vi "Save File DOE Reinitialize Drop Downs to Default.vi"(7 "Save Default":enum16{"Standard", "Save To Default"}(ring), 8 "error in (no error)":errorcluster, 11 "Standard Path":path=path "C:/GE/Washer DOE/WasherDOEConfig_Default.csv") -> (0 "error out":errorcluster, 3 "Default Data":string[][](array[string]))   [LabVIEW 2023, in "File Setup.lvlib"]
uses:
  File Setup.lvlib
  <vilib>/Utility/file.llb/Read From Spreadsheet File (string).vi
  <vilib>/Utility/file.llb/Write To Spreadsheet File (string).vi
panel:
  in  "Default Path":path=path "C:/GE/Washer DOE/WasherDOEConfig_Default.csv"
  # "Only change drop down menu items. Others include the \ncalibration data ect."
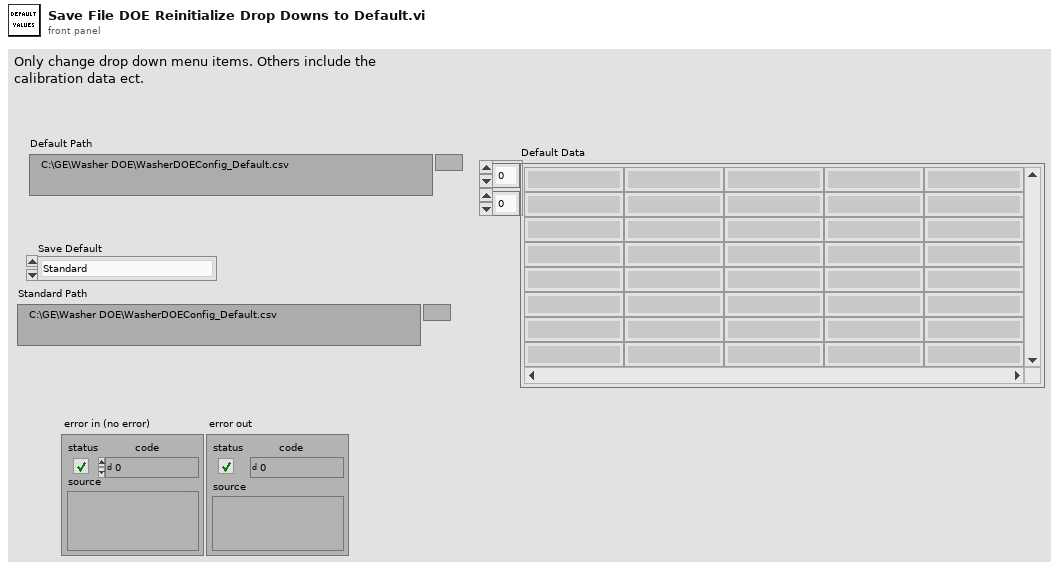
[diagram p1: front panel]
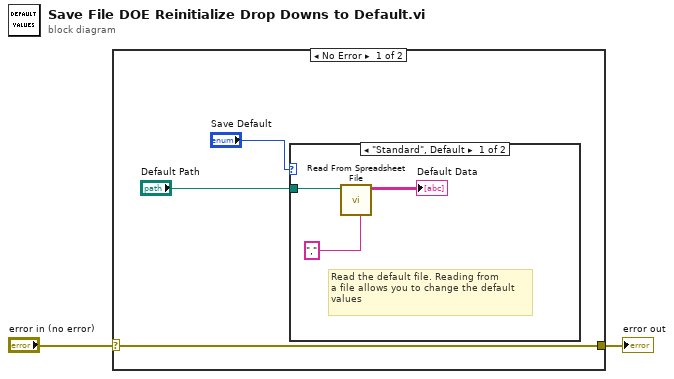
[diagram p0: block diagram]
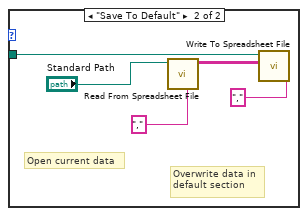
[diagram p2: hidden frame]
diagram:
  n1 = case shown="No Error" "error in (no error)" {
    selector: "error in (no error)" -> [w5 w14]
    tunnel: [w5 w14] -> w1
    frame No Error {
      n2 = case shown="\"Standard\", Default" "Save Default" {
        tunnel: "Default Path" -> [w6 w12]
        frame "Standard", Default {
          # "Read the default file. Reading from\na file allows you to change the default\nvalues"
          n3 = call-poly <vilib>:"Read From Spreadsheet File.vi"("delimiter (\\t)"="," ("delimiter (\\t)"), "file path (dialog if empty)"=w6) -> ("all rows"=→"Default Data":string[][])  [unwired: 5 in, 4 out]
        }
        frame "Save To Default" {
          # "Overwrite data in\ndefault section"
          # "Open current data"
          n4 = call-poly <vilib>:"Read From Spreadsheet File.vi"("delimiter (\\t)"="," ("delimiter (\\t)"), "file path (dialog if empty)"="Standard Path") -> ("all rows"=w11:string[][])  [unwired: 5 in, 4 out]
          n5 = call-poly <vilib>:"Write To Spreadsheet File.vi"("delimiter (\\t)"="," ("delimiter (\\t)"), "2D data"=w11, "file path (dialog if empty)"=w12) -> ()  [unwired: 5 in, 1 out]
        }
      }
    }
    frame Error {
    }
  }
  "error out" <- w1
